vi "Append to Array - Known Type.vi"(5 "JSON Compatible Type":T1=enum."Unknown", 6 "Add Parameter as JSON Tree?":bool, 7 "JSON Type":T2=enum."Unknown", 8 "error in (no error)":errorcluster, 10 "Value":variant, 11 "JSON Tree in (JSON Array)":variant) -> (0 "error out":errorcluster, 3 "JSON Tree out (JSON Array)":variant)   [LabVIEW 2011, in "i3-json.lvlib"]
doc: "Use this template to build a VI to use as a subVI."
uses:
  i3-json.lvlib
  JSON Types/JSON Type.ctl
  JSON Types/JSON Compatible Type.ctl
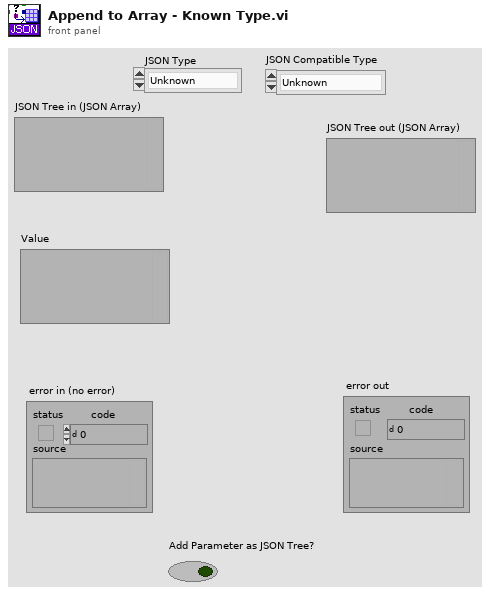
[diagram p1: front panel]
types:
  T1 = typedef "i3-json.lvlib/JSON Compatible Type.ctl" = enum16{"1D Double Array", "1D String Array", "1D Boolean Array", "Unknown"}
  T2 = typedef "i3-json.lvlib/JSON Type.ctl" = enum8{"JSON Compatible", "JSON Array", "JSON Object", "JSON Null", "Double", "String", "Boolean", "Unknown", "Data JSON string"}
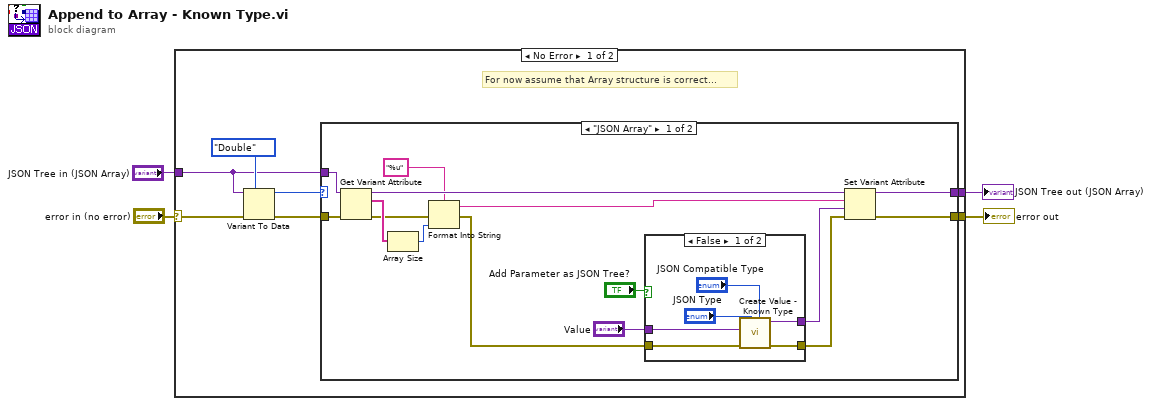
[diagram p0: block diagram]
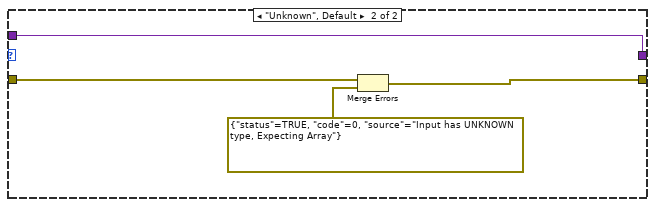
[diagram p3: hidden frame]
diagram:
  n1 = case shown="No Error" "error in (no error)" {
    selector: "error in (no error)" -> [w9 w40]
    tunnel: [w7 w40] -> w3
    tunnel: [w6 w39] -> w2
    tunnel: "JSON Tree in (JSON Array)" -> [w5 w39]
    frame No Error {
      # "For now assume that Array structure is correct..."
      n2 = Variant To Data(error in=w9, type=JSON_Type."Double" ("JSON Type"), Variant=w5) -> (data=w10:T2, error out=w8:errorcluster)
      n3 = case shown="\"JSON Array\"" w10 {
        tunnel: w5 -> [w25 w38]
        tunnel: w8 -> [w24 w37]
        tunnel: [w14 w38] -> w6
        tunnel: [w13 w36] -> w7
        frame "JSON Array" {
          n4 = Get Variant Attribute(Variant=w25, error in=w24) -> (duplicate Variant=w23:variant, names=w26:string[], error out=w20:errorcluster)  [unwired: 2 in, 1 out]
          n5 = Array Size(array=w26) -> (size(s)=w21:i32)
          n6 = Format Into String "Format Into String"(format string="%u", error in=w20, w21) -> (resulting string=w18:string, error out=w17:errorcluster)  [unwired: 1 in]
          n7 = case shown="False" "Add Parameter as JSON Tree?" {
            tunnel: "Value" -> [w30 w34]
            tunnel: w17 -> [w29 w33]
            tunnel: [w28 w33] -> w16
            tunnel: [w27 w34] -> w15
            frame False {
              n8 = call "Create Value - Known Type.vi"("JSON Compatible Type"="JSON Compatible Type", "JSON Type"="JSON Type", "error in (no error)"=w29, "Value"=w30) -> ("error out"=w28:errorcluster, "JSON Tree"=w27:variant)  [unwired: 6 in]
            }
            frame True {
              # "ASSUMES VALID\nJSON TREE - maybe\nshould run-time check?"
            }
          }
          n9 = Set Variant Attribute(Variant=w23, name=w18, value=w15, error in=w16) -> (Variant out=w14:variant, error out=w13:errorcluster)  [unwired: 1 out]
        }
        frame "Unknown", Default {
          n10 = Merge Errors(w37, errorcluster {"status"=TRUE, "code"=0, "source"="Input has UNKNOWN type, Expecting Array"} ("error in")) -> (w36:errorcluster)
        }
      }
    }
    frame Error {
    }
  }
  "error out" <- w3
  "JSON Tree out (JSON Array)" <- w2
